vi "Write Component Config File.vi"(8 "error in (no error)":errorcluster, 10 "Component Config File":path, 11 "Component in":refnum<class "Component.lvclass">) -> (0 "error out":errorcluster, 3 "Component out":refnum<class "Component.lvclass">)   [LabVIEW 2017, in "CL_G3_VIComponentBuilder.lvlib" / "Component.lvclass"]
uses:
  Component.lvclass
  Component.lvclass/Component.ctl
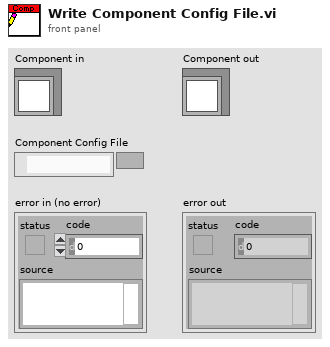
[diagram p1: front panel]
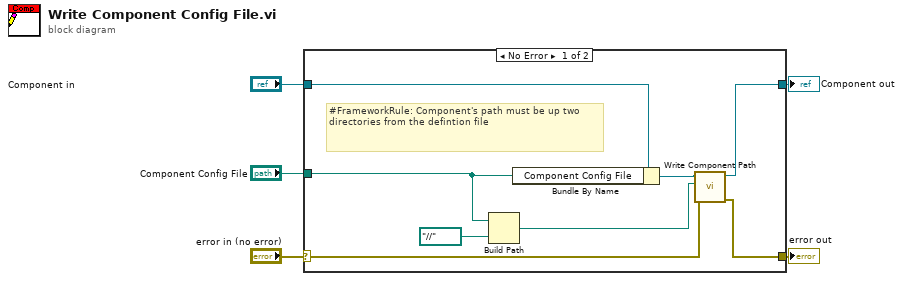
[diagram p0: block diagram]
diagram:
  n1 = case shown="No Error" "error in (no error)" {
    selector: "error in (no error)" -> [w7 w14]
    tunnel: [w6 w14] -> w4
    tunnel: [w8 w15] -> w2
    tunnel: "Component in" -> [w11 w15]
    tunnel: "Component Config File" -> [w12 _]
    frame No Error {
      # "#FrameworkRule: Component's path must be up two directories from the defintion file"
      n2 = Build Path(base path=w12, name or relative path=path "../../.." ("Accessors:Component Config File")) -> (appended path=w9:path)
      n3 = Bundle By Name(cluster=w11, "Component Config File"=w12) -> (w10:refnum<class "Component.lvclass">)
      n4 = call "Write Component Path.vi"("error in (no error)"=w7, "Component's Path"=w9, "Component in"=w10) -> ("error out"=w6:errorcluster, "Component out"=w8:refnum<class "Component.lvclass">)  [unwired: 7 in]
    }
    frame Error {
    }
  }
  "error out" <- w4
  "Component out" <- w2
